vi "ep_Check Spectra Settings.vi"(8 "error in (no error)":errorcluster, 10 "dt":dbl, 11 "spectra settings":T1={"number of lines"=12501, "% overlap"=0.0, "maximum frequency [Hz]"=250.0}) -> (0 "error out":errorcluster, 2 "fs":dbl, 3 "dup spectra settings":T1={"number of lines"=12501, "% overlap"=0.0, "maximum frequency [Hz]"=250.0})   [LabVIEW 2014, in "NI_EP_Motor Monitoring.lvlib"]
uses:
  <vilib>/addons/Electrical Power/Motor Monitoring/NI_EP_Motor Monitoring.lvlib
  <vilib>/addons/Electrical Power/Motor Monitoring/subVIs/ep_Spectra Settings.ctl
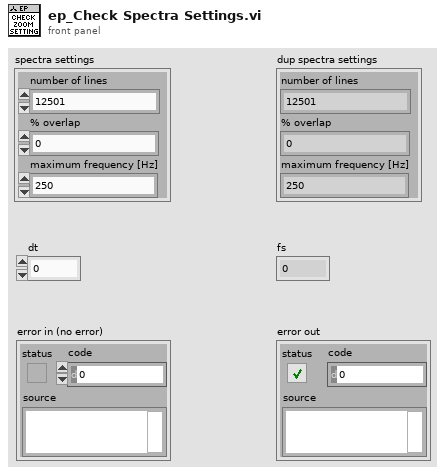
[diagram p1: front panel]
types:
  T1 = typedef "NI_EP_Motor Monitoring.lvlib/ep_Spectra Settings.ctl" = cluster{"number of lines":i32, "% overlap":dbl, "maximum frequency [Hz]":dbl}
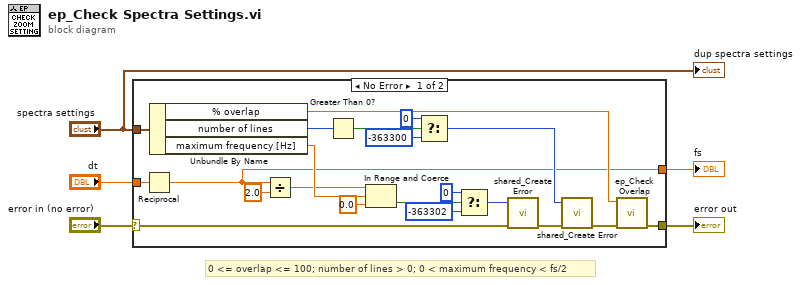
[diagram p0: block diagram]
diagram:
  # "0 <= overlap <= 100; number of lines > 0; 0 < maximum frequency < fs/2"
  n1 = case shown="No Error" "error in (no error)" {
    selector: "error in (no error)" -> [w26 w27]
    tunnel: "spectra settings" -> [w25 _]
    tunnel: "dt" -> [w24 _]
    tunnel: [w23 w27] -> w3
    tunnel: [w6 _] -> w2
    frame No Error {
      n2 = Reciprocal(x=w24) -> (1/x=w6:dbl)
      n3 = Unbundle By Name(w25) -> ("% overlap"=w9:dbl, "number of lines"=w10:i32, "maximum frequency [Hz]"=w14:dbl)
      n4 = Divide(x=w6, y=2.0) -> (x/y=w13:dbl)
      n5 = Greater Than 0?(x=w10) -> (x > 0?=w22:bool)
      n6 = In Range and Coerce(upper limit=w13, x=w14, lower limit=0.0) -> (In Range?=w18:bool)  [unwired: 1 out]
      n7 = Select(t=0 ("error code (0)"), s=w22, f=-363300 ("error code (0)")) -> (s? t:f=w19:i32)
      n8 = Select(t=0 ("error code (0)"), s=w18, f=-363302 ("error code (0)")) -> (s? t:f=w12:i32)
      n9 = call <vilib>:"shared_Create Error.vi"("error in (no error)"=w26, "error code (0)"=w12) -> ("error out"=w8:errorcluster)  [unwired: 9 in]
      n10 = call <vilib>:"shared_Create Error.vi"("error in (no error)"=w8, "error code (0)"=w19) -> ("error out"=w11:errorcluster)  [unwired: 9 in]
      n11 = call <vilib>:"ep_Check Overlap.vi"("error in (no error)"=w11, "% overlap"=w9) -> ("error out"=w23:errorcluster)  [unwired: 9 in]
    }
    frame Error {
    }
  }
  "error out" <- w3
  "fs" <- w2
  "dup spectra settings" <- "spectra settings"
